vi "HolDrvCtrl_Calculate.vi"(7 "currentPose":T3={"TRANSLATION"={"X"=0.0, "Y"=0.0}, "ROTATION"={"VALUE"=0.0, "COS"=1.0, "SIN"=0.0}} {"ROTATION"."SIN" format="%13.4f"; "ROTATION"."COS" format="%13.4f"; "ROTATION"."VALUE" format="%13.4f"; "TRANSLATION"."Y" format="%14.3f"; "TRANSLATION"."X" format="%14.3f"}, 8 "angleRef":T2={"VALUE"=0.0, "COS"=1.0, "SIN"=0.0} {"SIN" format="%13.4f"; "COS" format="%13.4f"; "VALUE" format="%13.4f"}, 9 "linearVelRef":dbl, 10 "poseRef":T3={"TRANSLATION"={"X"=0.0, "Y"=0.0}, "ROTATION"={"VALUE"=0.0, "COS"=1.0, "SIN"=0.0}} {"ROTATION"."SIN" format="%13.4f"; "ROTATION"."COS" format="%13.4f"; "ROTATION"."VALUE" format="%13.4f"; "TRANSLATION"."Y" format="%14.3f"; "TRANSLATION"."X" format="%14.3f"}, 11 "inHOLONOMIC_DRV_CTRL":T5={"poseTolerance"={"TRANSLATION"={"X"=0.0, "Y"=0.0}, "ROTATION"={"VALUE"=0.0, "COS"=1.0, "SIN"=0.0}}, "poseError"={"TRANSLATION"={"X"=0.0, "Y"=0.0}, "ROTATION"={"VALUE"=0.0, "COS"=1.0, "SIN"=0.0}}, "Enabled"=TRUE, "PID_xCtrl"={"Kp"=0.0, "Ki"=0.0, "Kd"=0.0, "Period"=0.0, "Max_Integral"=1.0, "Min_Integral"=-1.0, "Max_Input"=0.0, "Min_Input"=0.0, "Continuous"=FALSE, "PositionError"=0.0, "VelocityError"=0.0, "PrevError"=0.0, "TotalError"=0.0, "PositionTolerance"=0.05, "VelocityTolerance"=9.99e+35, "SetPoint"=0.0, "Kf"=0.0, "Prev_Deriv"=0.0, "Prev_Deriv 2"=0.0, "DerivativeFilter"=FALSE, "Min_Output"=-9.99e+35, "Max_Output"=9.9e+35, "Prev_F_P"=0.0, "Prev_F_P_2"=0.0, "AntiWindupActive"=FALSE}, "PID_yCtrl"={"Kp"=0.0, "Ki"=0.0, "Kd"=0.0, "Period"=0.0, "Max_Integral"=1.0, "Min_Integral"=-1.0, "Max_Input"=0.0, "Min_Input"=0.0, "Continuous"=FALSE, "PositionError"=0.0, "VelocityError"=0.0, "PrevError"=0.0, "TotalError"=0.0, "PositionTolerance"=0.05, "VelocityTolerance"=9.99e+35, "SetPoint"=0.0, "Kf"=0.0, "Prev_Deriv"=0.0, "Prev_Deriv 2"=0.0, "DerivativeFilter"=FALSE, "Min_Output"=-9.99e+35, "Max_Output"=9.9e+35, "Prev_F_P"=0.0, "Prev_F_P_2"=0.0, "AntiWindupActive"=FALSE}, "PROF_PID_thetaCtrl"={"Controller"={"Kp"=0.0, "Ki"=0.0, "Kd"=0.0, "Period"=0.0, "Max_Integral"=1.0, "Min_Integral"=-1.0, "Max_Input"=0.0, "Min_Input"=0.0, "Continuous"=FALSE, "PositionError"=0.0, "VelocityError"=0.0, "PrevError"=0.0, "TotalError"=0.0, "PositionTolerance"=0.05, "VelocityTolerance"=9.99e+35, "SetPoint"=0.0, "Kf"=0.0, "Prev_Deriv"=0.0, "Prev_Deriv 2"=0.0, "DerivativeFilter"=FALSE, "Min_Output"=-9.99e+35, "Max_Output"=9.9e+35, "Prev_F_P"=0.0, "Prev_F_P_2"=0.0, "AntiWindupActive"=FALSE}, "Goal"={"Position"=0.0, "Velocity"=0.0}, "Setpoint"={"Position"=0.0, "Velocity"=0.0}, "Constraint"={"MaxVelocity"=0.0, "MaxAcceleration"=0.0}}} {"PROF_PID_thetaCtrl"."Constraint"."MaxAcceleration" format="%16_6e"; "PROF_PID_thetaCtrl"."Constraint"."MaxVelocity" format="%16_6e"; "PROF_PID_thetaCtrl"."Setpoint"."Velocity" format="%16_6e"; "PROF_PID_thetaCtrl"."Setpoint"."Position" format="%16_6e"; "PROF_PID_thetaCtrl"."Goal"."Velocity" format="%16_6e"; "PROF_PID_thetaCtrl"."Goal"."Position" format="%16_6e"; "PROF_PID_thetaCtrl"."Controller"."Prev_F_P_2" format="%16_6e"; "PROF_PID_thetaCtrl"."Controller"."Prev_F_P" format="%16_6e"; "PROF_PID_thetaCtrl"."Controller"."Max_Output" format="%16_6e"; "PROF_PID_thetaCtrl"."Controller"."Min_Output" format="%16_6e"; "PROF_PID_thetaCtrl"."Controller"."Prev_Deriv 2" format="%16_6e"; "PROF_PID_thetaCtrl"."Controller"."Prev_Deriv" format="%16_6e"; "PROF_PID_thetaCtrl"."Controller"."Kf" format="%16_6e"; "PROF_PID_thetaCtrl"."Controller"."SetPoint" format="%16_6e"; "PROF_PID_thetaCtrl"."Controller"."VelocityTolerance" format="%16_6e"; "PROF_PID_thetaCtrl"."Controller"."PositionTolerance" format="%16_6e"; "PROF_PID_thetaCtrl"."Controller"."TotalError" format="%16_6e"; "PROF_PID_thetaCtrl"."Controller"."PrevError" format="%16_6e"; "PROF_PID_thetaCtrl"."Controller"."VelocityError" format="%16_6e"; "PROF_PID_thetaCtrl"."Controller"."PositionError" format="%16_6e"; "PROF_PID_thetaCtrl"."Controller"."Min_Input" format="%16_6e"; "PROF_PID_thetaCtrl"."Controller"."Max_Input" format="%16_6e"; "PROF_PID_thetaCtrl"."Controller"."Min_Integral" format="%16_6e"; "PROF_PID_thetaCtrl"."Controller"."Max_Integral" format="%16_6e"; "PROF_PID_thetaCtrl"."Controller"."Period" format="%16_6e"; "PROF_PID_thetaCtrl"."Controller"."Kd" format="%16_6e"; "PROF_PID_thetaCtrl"."Controller"."Ki" format="%16_6e"; "PROF_PID_thetaCtrl"."Controller"."Kp" format="%16_6e"; "PID_yCtrl"."Prev_F_P_2" format="%16_6e"; "PID_yCtrl"."Prev_F_P" format="%16_6e"; "PID_yCtrl"."Max_Output" format="%16_6e"; "PID_yCtrl"."Min_Output" format="%16_6e"; "PID_yCtrl"."Prev_Deriv 2" format="%16_6e"; "PID_yCtrl"."Prev_Deriv" format="%16_6e"; "PID_yCtrl"."Kf" format="%16_6e"; "PID_yCtrl"."SetPoint" format="%16_6e"; "PID_yCtrl"."VelocityTolerance" format="%16_6e"; "PID_yCtrl"."PositionTolerance" format="%16_6e"; "PID_yCtrl"."TotalError" format="%16_6e"; "PID_yCtrl"."PrevError" format="%16_6e"; "PID_yCtrl"."VelocityError" format="%16_6e"; "PID_yCtrl"."PositionError" format="%16_6e"; "PID_yCtrl"."Min_Input" format="%16_6e"; "PID_yCtrl"."Max_Input" format="%16_6e"; "PID_yCtrl"."Min_Integral" format="%16_6e"; "PID_yCtrl"."Max_Integral" format="%16_6e"; "PID_yCtrl"."Period" format="%16_6e"; "PID_yCtrl"."Kd" format="%16_6e"; "PID_yCtrl"."Ki" format="%16_6e"; "PID_yCtrl"."Kp" format="%16_6e"; "PID_xCtrl"."Prev_F_P_2" format="%16_6e"; "PID_xCtrl"."Prev_F_P" format="%16_6e"; "PID_xCtrl"."Max_Output" format="%16_6e"; "PID_xCtrl"."Min_Output" format="%16_6e"; "PID_xCtrl"."Prev_Deriv 2" format="%16_6e"; "PID_xCtrl"."Prev_Deriv" format="%16_6e"; "PID_xCtrl"."Kf" format="%16_6e"; "PID_xCtrl"."SetPoint" format="%16_6e"; "PID_xCtrl"."VelocityTolerance" format="%16_6e"; "PID_xCtrl"."PositionTolerance" format="%16_6e"; "PID_xCtrl"."TotalError" format="%16_6e"; "PID_xCtrl"."PrevError" format="%16_6e"; "PID_xCtrl"."VelocityError" format="%16_6e"; "PID_xCtrl"."PositionError" format="%16_6e"; "PID_xCtrl"."Min_Input" format="%16_6e"; "PID_xCtrl"."Max_Input" format="%16_6e"; "PID_xCtrl"."Min_Integral" format="%16_6e"; "PID_xCtrl"."Max_Integral" format="%16_6e"; "PID_xCtrl"."Period" format="%16_6e"; "PID_xCtrl"."Kd" format="%16_6e"; "PID_xCtrl"."Ki" format="%16_6e"; "PID_xCtrl"."Kp" format="%16_6e"; "poseError"."ROTATION"."SIN" format="%13.4f"; "poseError"."ROTATION"."COS" format="%13.4f"; "poseError"."ROTATION"."VALUE" format="%13.4f"; "poseError"."TRANSLATION"."Y" format="%14.3f"; "poseError"."TRANSLATION"."X" format="%14.3f"; "poseTolerance"."ROTATION"."SIN" format="%13.4f"; "poseTolerance"."ROTATION"."COS" format="%13.4f"; "poseTolerance"."ROTATION"."VALUE" format="%13.4f"; "poseTolerance"."TRANSLATION"."Y" format="%14.3f"; "poseTolerance"."TRANSLATION"."X" format="%14.3f"}) -> (1 "calcChassisSpeed":T1 {"vOmega" format="%10.3f"; "vY" format="%10.3f"; "vX" format="%10.3f"}, 3 "outHOLONOMIC_DRV_CTRL":T5={"poseTolerance"={"TRANSLATION"={"X"=0.0, "Y"=0.0}, "ROTATION"={"VALUE"=0.0, "COS"=1.0, "SIN"=0.0}}, "poseError"={"TRANSLATION"={"X"=0.0, "Y"=0.0}, "ROTATION"={"VALUE"=0.0, "COS"=1.0, "SIN"=0.0}}, "Enabled"=TRUE, "PID_xCtrl"={"Kp"=0.0, "Ki"=0.0, "Kd"=0.0, "Period"=0.0, "Max_Integral"=1.0, "Min_Integral"=-1.0, "Max_Input"=0.0, "Min_Input"=0.0, "Continuous"=FALSE, "PositionError"=0.0, "VelocityError"=0.0, "PrevError"=0.0, "TotalError"=0.0, "PositionTolerance"=0.05, "VelocityTolerance"=9.99e+35, "SetPoint"=0.0, "Kf"=0.0, "Prev_Deriv"=0.0, "Prev_Deriv 2"=0.0, "DerivativeFilter"=FALSE, "Min_Output"=-9.99e+35, "Max_Output"=9.9e+35, "Prev_F_P"=0.0, "Prev_F_P_2"=0.0, "AntiWindupActive"=FALSE}, "PID_yCtrl"={"Kp"=0.0, "Ki"=0.0, "Kd"=0.0, "Period"=0.0, "Max_Integral"=1.0, "Min_Integral"=-1.0, "Max_Input"=0.0, "Min_Input"=0.0, "Continuous"=FALSE, "PositionError"=0.0, "VelocityError"=0.0, "PrevError"=0.0, "TotalError"=0.0, "PositionTolerance"=0.05, "VelocityTolerance"=9.99e+35, "SetPoint"=0.0, "Kf"=0.0, "Prev_Deriv"=0.0, "Prev_Deriv 2"=0.0, "DerivativeFilter"=FALSE, "Min_Output"=-9.99e+35, "Max_Output"=9.9e+35, "Prev_F_P"=0.0, "Prev_F_P_2"=0.0, "AntiWindupActive"=FALSE}, "PROF_PID_thetaCtrl"={"Controller"={"Kp"=0.0, "Ki"=0.0, "Kd"=0.0, "Period"=0.0, "Max_Integral"=1.0, "Min_Integral"=-1.0, "Max_Input"=0.0, "Min_Input"=0.0, "Continuous"=FALSE, "PositionError"=0.0, "VelocityError"=0.0, "PrevError"=0.0, "TotalError"=0.0, "PositionTolerance"=0.05, "VelocityTolerance"=9.99e+35, "SetPoint"=0.0, "Kf"=0.0, "Prev_Deriv"=0.0, "Prev_Deriv 2"=0.0, "DerivativeFilter"=FALSE, "Min_Output"=-9.99e+35, "Max_Output"=9.9e+35, "Prev_F_P"=0.0, "Prev_F_P_2"=0.0, "AntiWindupActive"=FALSE}, "Goal"={"Position"=0.0, "Velocity"=0.0}, "Setpoint"={"Position"=0.0, "Velocity"=0.0}, "Constraint"={"MaxVelocity"=0.0, "MaxAcceleration"=0.0}}} {"PROF_PID_thetaCtrl"."Constraint"."MaxAcceleration" format="%16_6e"; "PROF_PID_thetaCtrl"."Constraint"."MaxVelocity" format="%16_6e"; "PROF_PID_thetaCtrl"."Setpoint"."Velocity" format="%16_6e"; "PROF_PID_thetaCtrl"."Setpoint"."Position" format="%16_6e"; "PROF_PID_thetaCtrl"."Goal"."Velocity" format="%16_6e"; "PROF_PID_thetaCtrl"."Goal"."Position" format="%16_6e"; "PROF_PID_thetaCtrl"."Controller"."Prev_F_P_2" format="%16_6e"; "PROF_PID_thetaCtrl"."Controller"."Prev_F_P" format="%16_6e"; "PROF_PID_thetaCtrl"."Controller"."Max_Output" format="%16_6e"; "PROF_PID_thetaCtrl"."Controller"."Min_Output" format="%16_6e"; "PROF_PID_thetaCtrl"."Controller"."Prev_Deriv 2" format="%16_6e"; "PROF_PID_thetaCtrl"."Controller"."Prev_Deriv" format="%16_6e"; "PROF_PID_thetaCtrl"."Controller"."Kf" format="%16_6e"; "PROF_PID_thetaCtrl"."Controller"."SetPoint" format="%16_6e"; "PROF_PID_thetaCtrl"."Controller"."VelocityTolerance" format="%16_6e"; "PROF_PID_thetaCtrl"."Controller"."PositionTolerance" format="%16_6e"; "PROF_PID_thetaCtrl"."Controller"."TotalError" format="%16_6e"; "PROF_PID_thetaCtrl"."Controller"."PrevError" format="%16_6e"; "PROF_PID_thetaCtrl"."Controller"."VelocityError" format="%16_6e"; "PROF_PID_thetaCtrl"."Controller"."PositionError" format="%16_6e"; "PROF_PID_thetaCtrl"."Controller"."Min_Input" format="%16_6e"; "PROF_PID_thetaCtrl"."Controller"."Max_Input" format="%16_6e"; "PROF_PID_thetaCtrl"."Controller"."Min_Integral" format="%16_6e"; "PROF_PID_thetaCtrl"."Controller"."Max_Integral" format="%16_6e"; "PROF_PID_thetaCtrl"."Controller"."Period" format="%16_6e"; "PROF_PID_thetaCtrl"."Controller"."Kd" format="%16_6e"; "PROF_PID_thetaCtrl"."Controller"."Ki" format="%16_6e"; "PROF_PID_thetaCtrl"."Controller"."Kp" format="%16_6e"; "PID_yCtrl"."Prev_F_P_2" format="%16_6e"; "PID_yCtrl"."Prev_F_P" format="%16_6e"; "PID_yCtrl"."Max_Output" format="%16_6e"; "PID_yCtrl"."Min_Output" format="%16_6e"; "PID_yCtrl"."Prev_Deriv 2" format="%16_6e"; "PID_yCtrl"."Prev_Deriv" format="%16_6e"; "PID_yCtrl"."Kf" format="%16_6e"; "PID_yCtrl"."SetPoint" format="%16_6e"; "PID_yCtrl"."VelocityTolerance" format="%16_6e"; "PID_yCtrl"."PositionTolerance" format="%16_6e"; "PID_yCtrl"."TotalError" format="%16_6e"; "PID_yCtrl"."PrevError" format="%16_6e"; "PID_yCtrl"."VelocityError" format="%16_6e"; "PID_yCtrl"."PositionError" format="%16_6e"; "PID_yCtrl"."Min_Input" format="%16_6e"; "PID_yCtrl"."Max_Input" format="%16_6e"; "PID_yCtrl"."Min_Integral" format="%16_6e"; "PID_yCtrl"."Max_Integral" format="%16_6e"; "PID_yCtrl"."Period" format="%16_6e"; "PID_yCtrl"."Kd" format="%16_6e"; "PID_yCtrl"."Ki" format="%16_6e"; "PID_yCtrl"."Kp" format="%16_6e"; "PID_xCtrl"."Prev_F_P_2" format="%16_6e"; "PID_xCtrl"."Prev_F_P" format="%16_6e"; "PID_xCtrl"."Max_Output" format="%16_6e"; "PID_xCtrl"."Min_Output" format="%16_6e"; "PID_xCtrl"."Prev_Deriv 2" format="%16_6e"; "PID_xCtrl"."Prev_Deriv" format="%16_6e"; "PID_xCtrl"."Kf" format="%16_6e"; "PID_xCtrl"."SetPoint" format="%16_6e"; "PID_xCtrl"."VelocityTolerance" format="%16_6e"; "PID_xCtrl"."PositionTolerance" format="%16_6e"; "PID_xCtrl"."TotalError" format="%16_6e"; "PID_xCtrl"."PrevError" format="%16_6e"; "PID_xCtrl"."VelocityError" format="%16_6e"; "PID_xCtrl"."PositionError" format="%16_6e"; "PID_xCtrl"."Min_Input" format="%16_6e"; "PID_xCtrl"."Max_Input" format="%16_6e"; "PID_xCtrl"."Min_Integral" format="%16_6e"; "PID_xCtrl"."Max_Integral" format="%16_6e"; "PID_xCtrl"."Period" format="%16_6e"; "PID_xCtrl"."Kd" format="%16_6e"; "PID_xCtrl"."Ki" format="%16_6e"; "PID_xCtrl"."Kp" format="%16_6e"; "poseError"."ROTATION"."SIN" format="%13.4f"; "poseError"."ROTATION"."COS" format="%13.4f"; "poseError"."ROTATION"."VALUE" format="%13.4f"; "poseError"."TRANSLATION"."Y" format="%14.3f"; "poseError"."TRANSLATION"."X" format="%14.3f"; "poseTolerance"."ROTATION"."SIN" format="%13.4f"; "poseTolerance"."ROTATION"."COS" format="%13.4f"; "poseTolerance"."ROTATION"."VALUE" format="%13.4f"; "poseTolerance"."TRANSLATION"."Y" format="%14.3f"; "poseTolerance"."TRANSLATION"."X" format="%14.3f"})   [LabVIEW 2019, in "Trajectory_Library.lvlib"]
doc: "Returns true if the pose error is within tolerance of the reference.\n\nParameters:\n -Holonomic_Drv_Ctrl - Holonomic_Drv_Ctrl data structure\n\nReturns:\n - At Reference - Return value"
uses:
  Trajectory_Library.lvlib
  TRANSLATION2D.ctl
  ROTATION2D.ctl
  POSE2D.ctl
  PID_CONTROLLER.ctl
  TRAPEZOID_PROFILE_STATE.ctl
  TRAPEZOID_PROFILE_CONSTRAINT.ctl
  PROFILED_PID_CONTROLLER.ctl
  HOLONOMIC_DRV_CTRL.ctl
  CHASSIS_SPEEDS.ctl
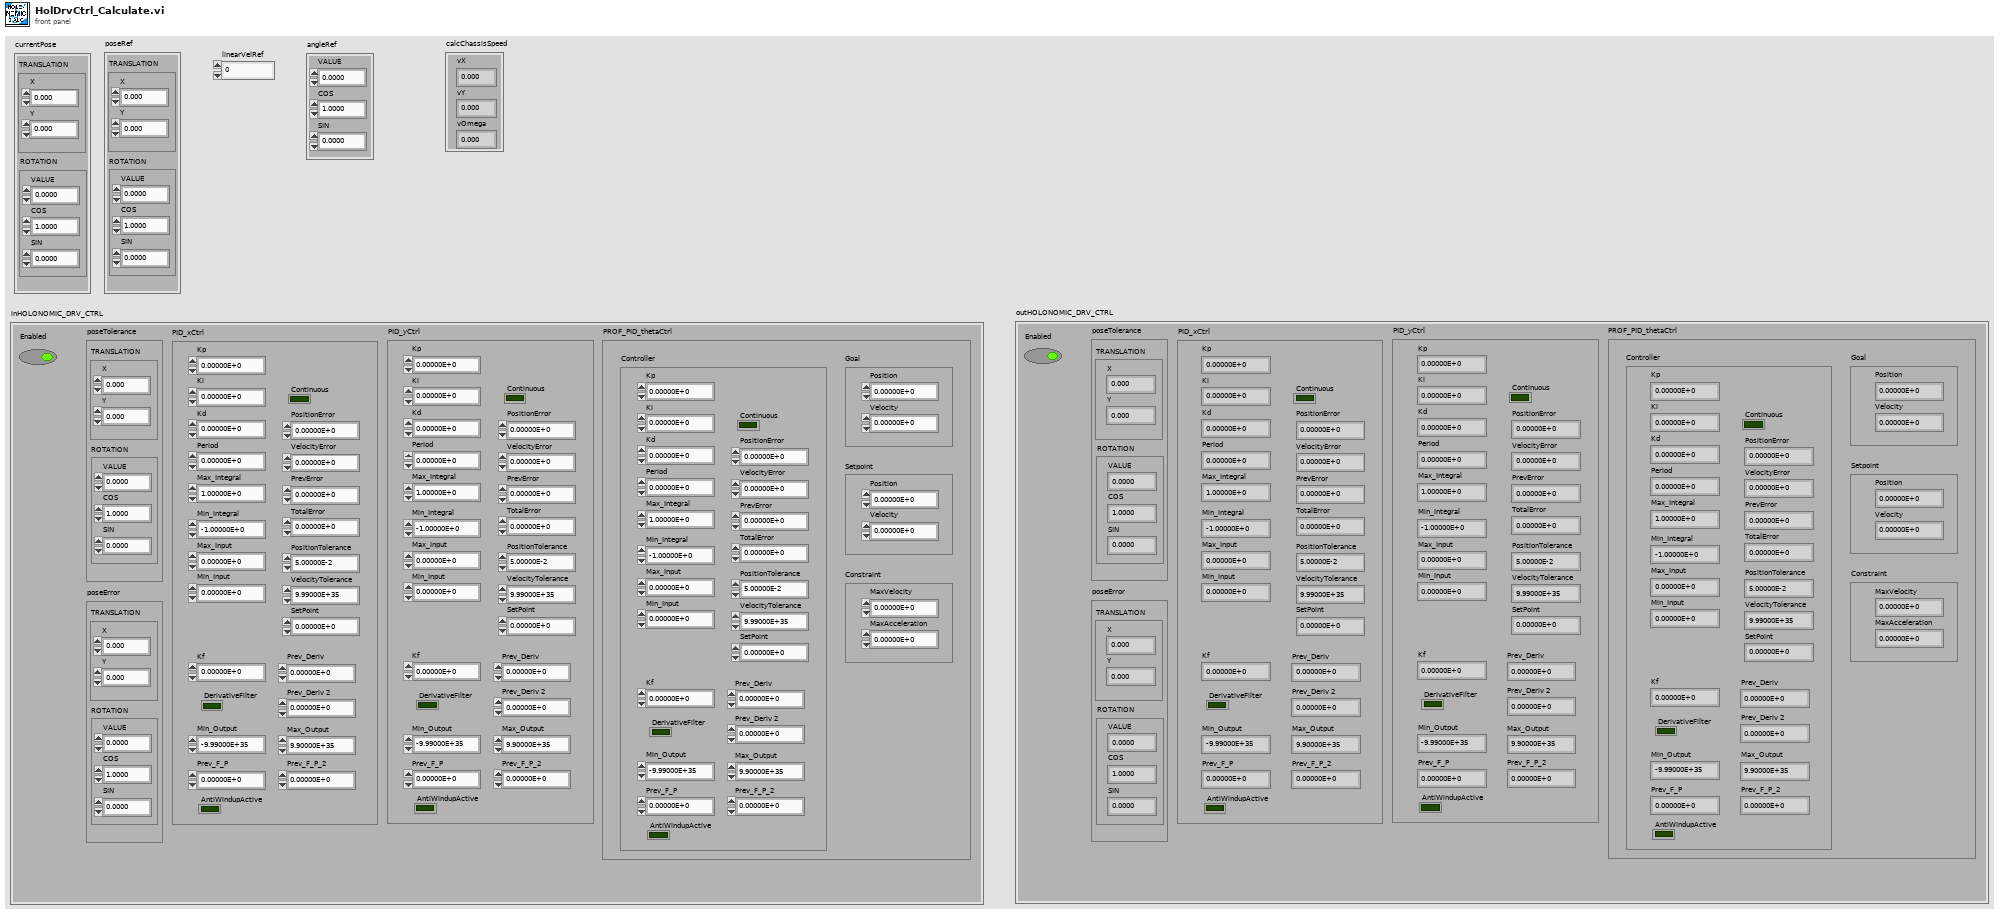
[diagram p1: front panel]
types:
  T1 = typedef "Trajectory_Library.lvlib/CHASSIS_SPEEDS.ctl" = cluster{"vX":dbl, "vY":dbl, "vOmega":dbl}
  T2 = typedef "Trajectory_Library.lvlib/ROTATION2D.ctl" = cluster{"VALUE":dbl, "COS":dbl, "SIN":dbl}
  T3 = typedef "Trajectory_Library.lvlib/POSE2D.ctl" = cluster{"TRANSLATION":T4, "ROTATION":T2}
  T4 = typedef "Trajectory_Library.lvlib/TRANSLATION2D.ctl" = cluster{"X":dbl, "Y":dbl}
  T5 = typedef "Trajectory_Library.lvlib/HOLONOMIC_DRV_CTRL.ctl" = cluster{"poseTolerance":T3, "poseError":T3, "Enabled":bool, "PID_xCtrl":T6, "PID_yCtrl":T6, "PROF_PID_thetaCtrl":T7}
  T6 = typedef "Trajectory_Library.lvlib/PID_CONTROLLER.ctl" = cluster{"Kp":dbl, "Ki":dbl, "Kd":dbl, "Period":dbl, "Max_Integral":dbl, "Min_Integral":dbl, "Max_Input":dbl, "Min_Input":dbl, "Continuous":bool, "PositionError":dbl, "VelocityError":dbl, "PrevError":dbl, "TotalError":dbl, "PositionTolerance":dbl, "VelocityTolerance":dbl, "SetPoint":dbl, "Kf":dbl, "Prev_Deriv":dbl, "Prev_Deriv 2":dbl, "DerivativeFilter":bool, "Min_Output":dbl, "Max_Output":dbl, "Prev_F_P":dbl, "Prev_F_P_2":dbl, "AntiWindupActive":bool}
  T7 = typedef "Trajectory_Library.lvlib/PROFILED_PID_CONTROLLER.ctl" = cluster{"Controller":T6, "Goal":T8, "Setpoint":T8, "Constraint":T9}
  T8 = typedef "Trajectory_Library.lvlib/TRAPEZOID_PROFILE_STATE.ctl" = cluster{"Position":dbl, "Velocity":dbl}
  T9 = typedef "Trajectory_Library.lvlib/TRAPEZOID_PROFILE_CONSTRAINT.ctl" = cluster{"MaxVelocity":dbl, "MaxAcceleration":dbl}
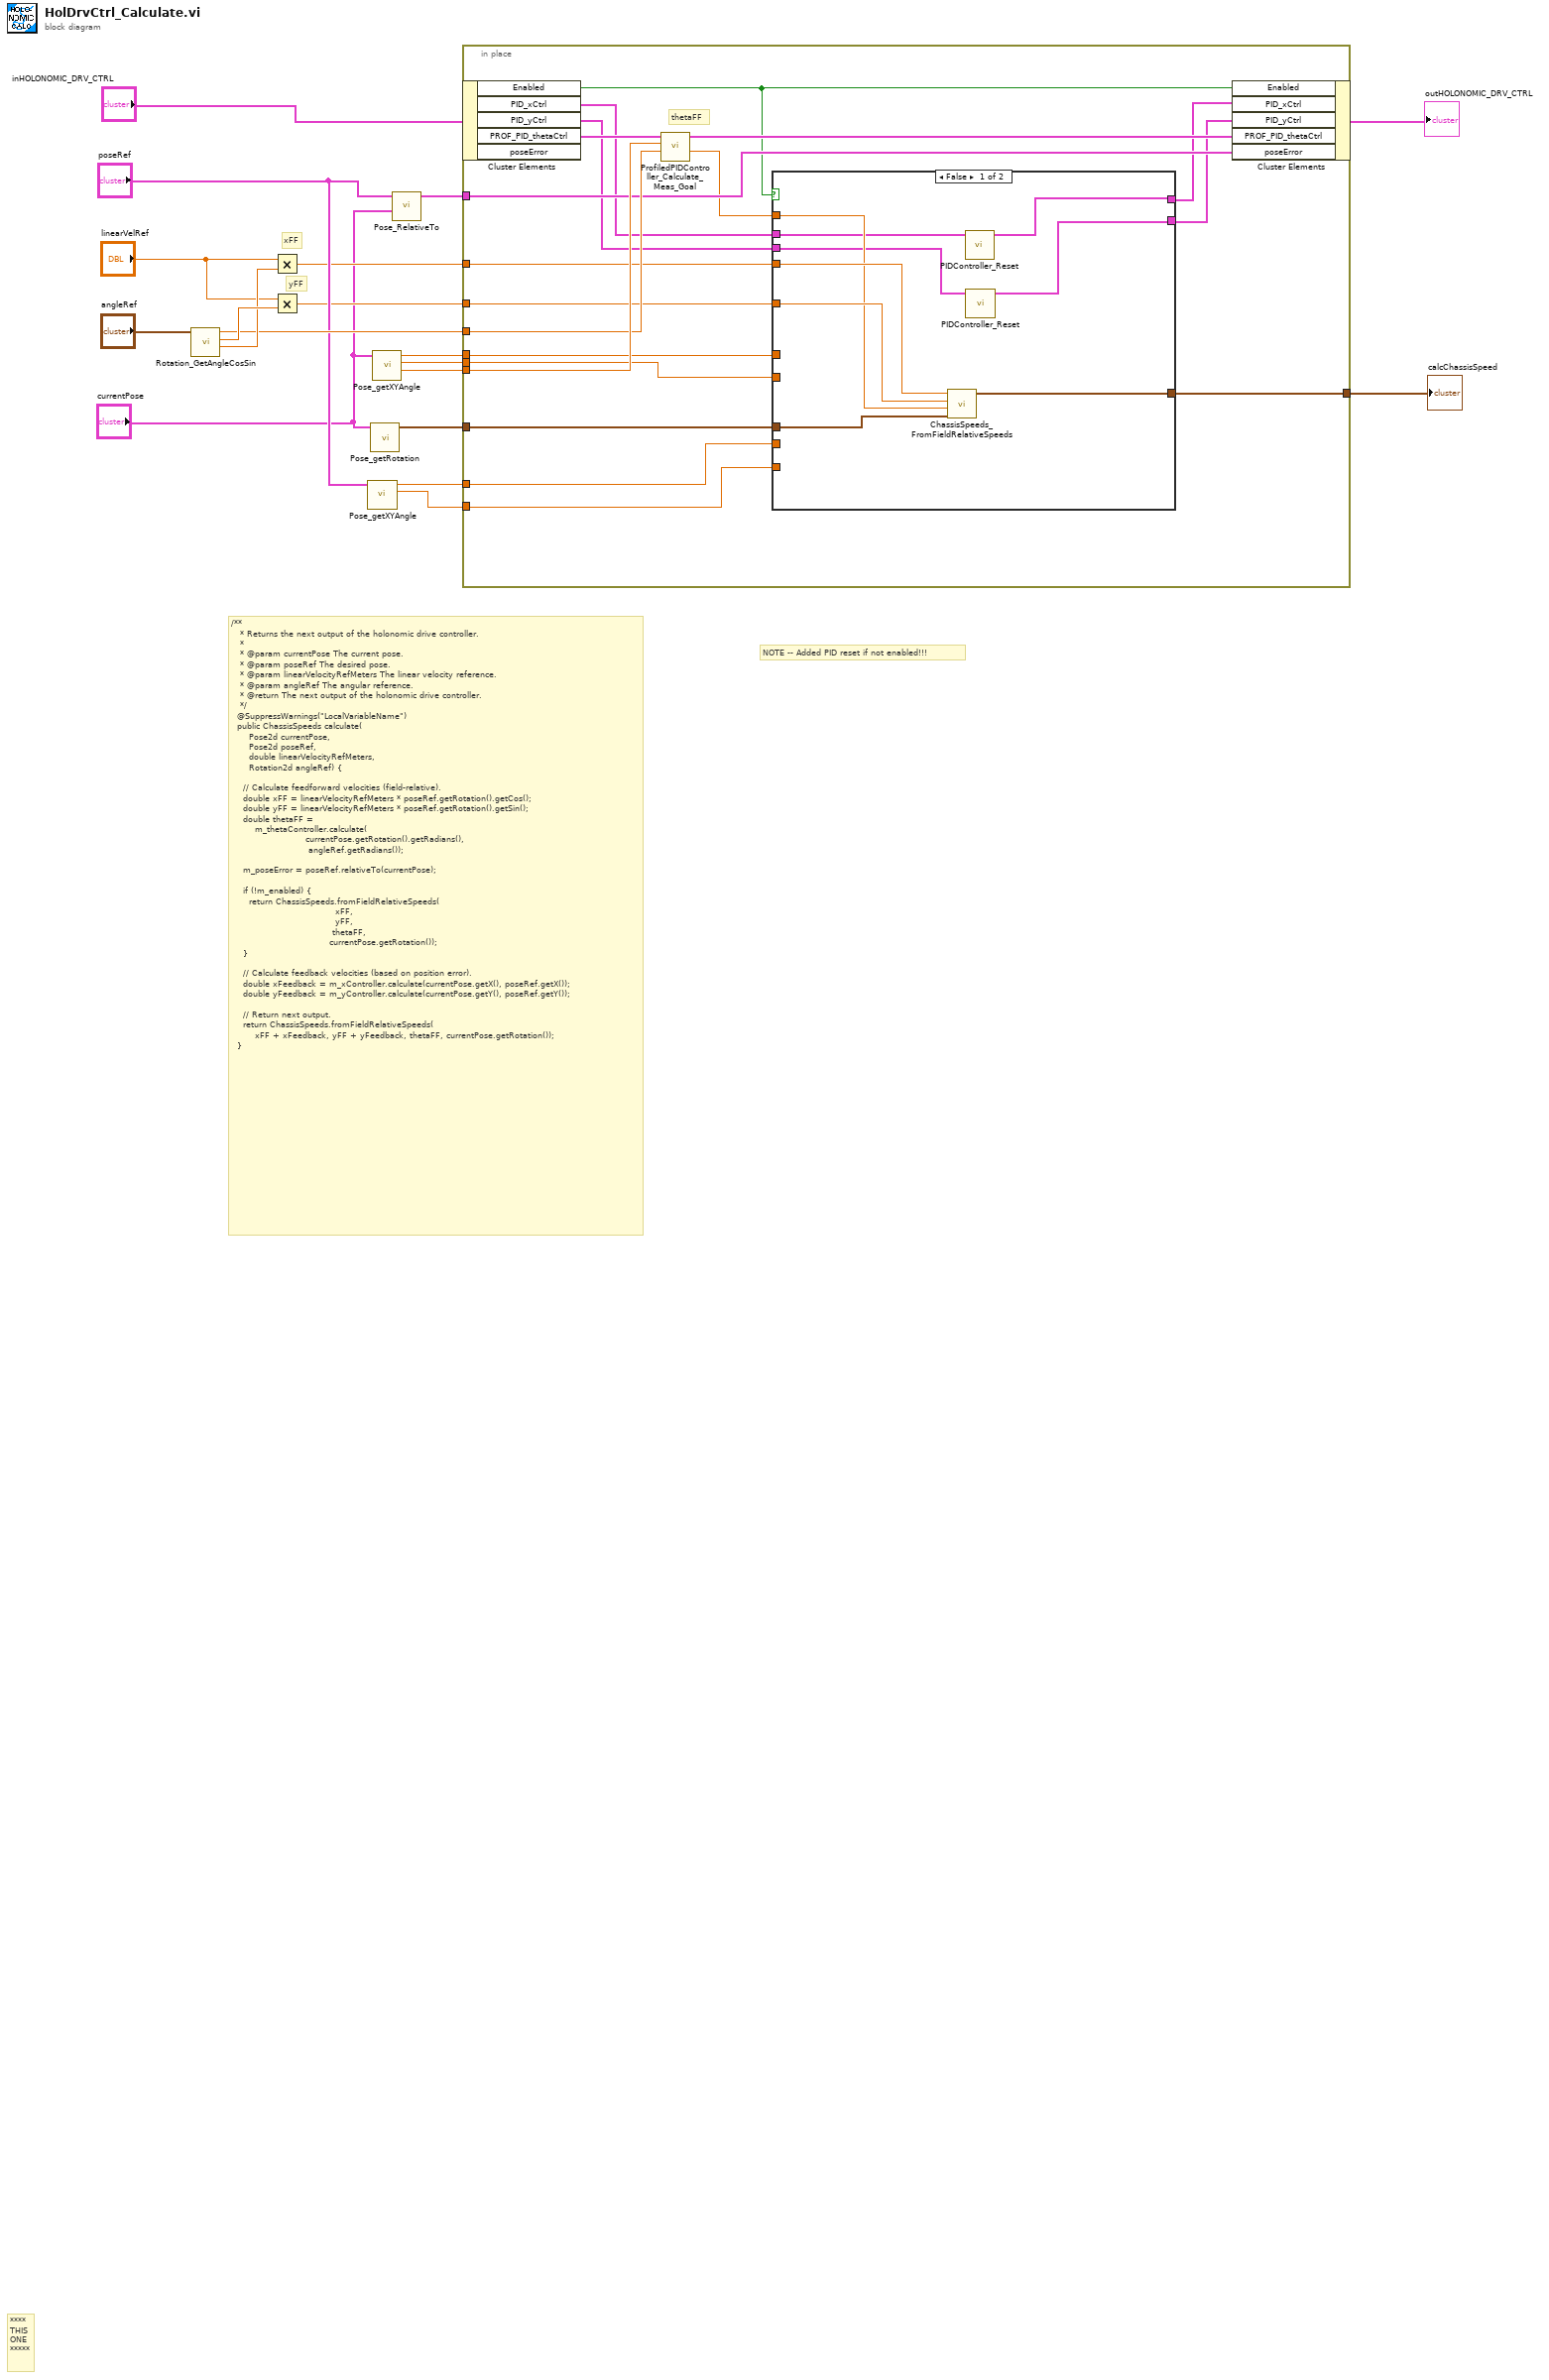
[diagram p0: block diagram]
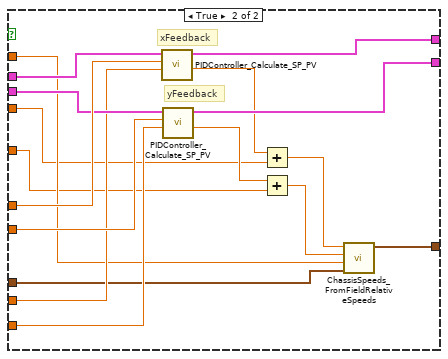
[diagram p2: hidden frame]
diagram:
  # "NOTE -- Added PID reset if not enabled!!!"
  # "yFF"
  # "xFF"
  # "****\nTHIS\nONE\n*****"
  # "/**\n   * Returns the next output of the holonomic drive controller.\n   *\n   * @param currentPose The current pose.\n   * @param poseRef The desired pose.\n   * @param linearVelocityRefMeters The linear velocity reference.\n   * @param angleRef The angular reference.\n   * @return The next output of the holonomic drive controller.\n   */\n  @SuppressWarnings(\"LocalVariableName\")\n  public ChassisSpeeds calculate(\n      Pose2d currentPose, \n      Pose2d poseRef, \n      double linearVelocityRefMeters, \n      Rotation2d angleRef) {\n\n    // Calculate feedforward velocities (field-relative).\n    double xFF = linearVelocityRefMeters * poseRef.getRotation().getCos();\n    double yFF = linearVelocityRefMeters * poseRef.getRotation().getSin();\n    double thetaFF =\n        m_thetaController.calculate(\n                         currentPose.getRotation().getRadians(), \n                          angleRef.getRadians());\n\n    m_poseError = poseRef.relativeTo(currentPose);\n\n    if (!m_enabled) {\n      return ChassisSpeeds.fromFieldRelativeSpeeds(\n                                   xFF, \n                                   yFF, \n                                  thetaFF, \n                                 currentPose.getRotation());\n    }\n\n    // Calculate feedback velocities (based on position error).\n    double xFeedback = m_xController.calculate(currentPose.getX(), poseRef.getX());\n    double yFeedback = m_yController.calculate(currentPose.getY(), poseRef.getY());\n\n    // Return next output.\n    return ChassisSpeeds.fromFieldRelativeSpeeds(\n        xFF + xFeedback, yFF + yFeedback, thetaFF, currentPose.getRotation());\n  }"
  n1 = call "Rotation_GetAngleCosSin.vi"("in ROTATION"="angleRef") -> ("Cosine"=w15:dbl, "Sine"=w16:dbl, "Angle"=w12:dbl)  [unwired: 8 in]
  n2 = Multiply(x="linearVelRef", y=w15) -> (x*y=w9:dbl)
  n3 = Multiply(x="linearVelRef", y=w16) -> (x*y=w8:dbl)
  n4 = call "Pose_getXYAngle.vi"("in POSE"="poseRef") -> ("Y"=w1:dbl, "X"=w2:dbl)  [unwired: 8 in, 1 out]
  n5 = call "Pose_getRotation.vi"("in POSE"="currentPose") -> ("out ROTATION"=w6:T2)  [unwired: 10 in]
  n6 = call "Pose_getXYAngle.vi"("in POSE"="currentPose") -> ("Angle"=w13:dbl, "Y"=w3:dbl, "X"=w4:dbl)  [unwired: 8 in]
  n7 = call "Pose_RelativeTo.vi"("other POSE"="currentPose", "in POSE"="poseRef") -> ("out POSE"=w10:T3)  [unwired: 9 in]
  n8 = in-place {
    in-place-border: w13 -> [w37]
    in-place-border: w12 -> [w36]
    in-place-border: w10 -> [w34]
    in-place-border: w9 -> [w33]
    in-place-border: w8 -> [w32]
    in-place-border: w6 -> [w30]
    in-place-border: [w29] -> w5
    in-place-border: w4 -> [w28]
    in-place-border: w3 -> [w25]
    in-place-border: w2 -> [w24]
    in-place-border: w1 -> [w23]
    # "thetaFF"
    n9 = in-place-cluster #1("inHOLONOMIC_DRV_CTRL") -> ("Enabled"=w22:bool, "PID_xCtrl"=w27:T6, "PID_yCtrl"=w26:T6, "PROF_PID_thetaCtrl"=w38:T7)  [unwired: 1 out]
    n10 = call "ProfiledPIDController_Calculate_Meas_Goal.vi"("SP-Goal"=w36, "PV-Measurement"=w37, "in PROFILED_PID_CONTROLLER"=w38) -> ("CO-ControlOutput"=w31:dbl, "out PROFILED_PID_CONTROLLER"=w35:T7)  [unwired: 7 in]
    n11 = case shown="False" w22 {
      tunnel: w33 -> [w47 w49]
      tunnel: w32 -> [w46 w48]
      tunnel: w31 -> [w45 w54]
      tunnel: w30 -> [w44 w55]
      tunnel: [w43 w56] -> w29
      tunnel: w28 -> [_ w64]
      tunnel: w27 -> [w42 w63]
      tunnel: w26 -> [w40 w62]
      tunnel: w25 -> [_ w61]
      tunnel: w24 -> [_ w60]
      tunnel: w23 -> [_ w59]
      tunnel: [w41 w58] -> w21
      tunnel: [w39 w57] -> w20
      frame False {
        n12 = call "ChassisSpeeds_FromFieldRelativeSpeeds.vi"("RobotAngle"=w44, "Omega"=w45, "vY"=w46, "vX"=w47) -> ("CHASSIS"=w43:T1)  [unwired: 7 in]
        n13 = call "PIDController_Reset.vi"("in PID_CONTROLLER"=w42) -> ("out PID_CONTROLLER"=w41:T6)  [unwired: 10 in]
        n14 = call "PIDController_Reset.vi"("in PID_CONTROLLER"=w40) -> ("out PID_CONTROLLER"=w39:T6)  [unwired: 10 in]
      }
      frame True {
        # "yFeedback"
        # "xFeedback"
        n15 = call "PIDController_Calculate_SP_PV.vi"("SP-SetPoint"=w60, "PV-Measurement"=w64, "in PID_CONTROLLER"=w63) -> ("CO-ControlOutput"=w51:dbl, "out PID_CONTROLLER"=w58:T6)  [unwired: 7 in]
        n16 = call "PIDController_Calculate_SP_PV.vi"("SP-SetPoint"=w59, "PV-Measurement"=w61, "in PID_CONTROLLER"=w62) -> ("CO-ControlOutput"=w50:dbl, "out PID_CONTROLLER"=w57:T6)  [unwired: 7 in]
        n17 = Add(x=w51, y=w49) -> (x+y=w52:dbl)
        n18 = Add(x=w50, y=w48) -> (x+y=w53:dbl)
        n19 = call "ChassisSpeeds_FromFieldRelativeSpeeds.vi"("RobotAngle"=w55, "Omega"=w54, "vY"=w53, "vX"=w52) -> ("CHASSIS"=w56:T1)  [unwired: 7 in]
      }
    }
    n20 = in-place-cluster #1("Enabled"=w22, "PID_xCtrl"=w21, "PID_yCtrl"=w20, "PROF_PID_thetaCtrl"=w35, "poseError"=w34) -> (→"outHOLONOMIC_DRV_CTRL":T5)
  }
  "calcChassisSpeed" <- w5
